vi "子界面-查看某框和报告生成.vi"(0 "框号":dbl format="%#_13g", 1 "框组":T4(array[cluster]), 2 "反射图":T1(plugin-control), 4 "标注图":T1(plugin-control)) -> ()   [LabVIEW 2018]
uses:
  <vilib>/vision/NI_Vision_Development_Module.lvlib
panel:
  out "反射图ROI对应区域灰度表":u32[](graph)
  out "报告生成路径":path
  out "?":T1(plugin-control)
  out "Threshold Image":T1(plugin-control)
  in  "格式字符串 2":string="%f"
  in  "分隔符（'\\'代码显示）":string="\t"
  out "分层测量结果":dbl[][](array[numeric]) format="%.2f"
  out "分层类检测结果":string[][](table)
  out "Threshold Image":T1(plugin-control)
  out "Threshold Image":T1(plugin-control)
  out "缺陷分类的临界值":sgl
  out "反射图ROI的最大灰度值":sgl
  in  "返回 2":bool
  in  "报告生成":bool
  in  "反射法图像-面积阈值设置":T3(array[cluster]) {"Measurement Parameter" items=["Area"]; "下限" min=0 step=1; "上限" min=0 step=1}
  in  "穿透法图像-灰度阈值设置":cluster{"下限":dbl, "下限":dbl}(slide)={"下限"=0.0, "下限"=65.10638427734375} scale=0.0..255.0
  in  "保存结果":bool
  in  "部位":string
  in  "Color":u32[](array[colorbox])=[3381759, 16776770, 16777225, 6618880]
  in  "Overlay Type":u16[](array[ring])=[2, 1, 3, 0] items=["Rectangle", "Numbers", "Points", "Lines"]
  in  "Tab Control":T5
  out "穿透ROI":T1(plugin-control)
  out "Threshold Image":T1(plugin-control)
  out "?":T1(plugin-control)
  out "?":T1(plugin-control)
  out "Threshold Image":T1(plugin-control)
  out "Threshold Image":T1(plugin-control)
  out "弥散测量结果":dbl[][](array[numeric]) format="%.2f"
  in  "产品序号":string
  in  "测试人":string
  in  "分隔符（'\\'代码显示）":string="\t"
  in  "格式字符串":string="%f"
  out "弥散类检测结果":string[][](table)
  out "?":string
  out "面积 (pixels)":i32
  # "所选区域信息"
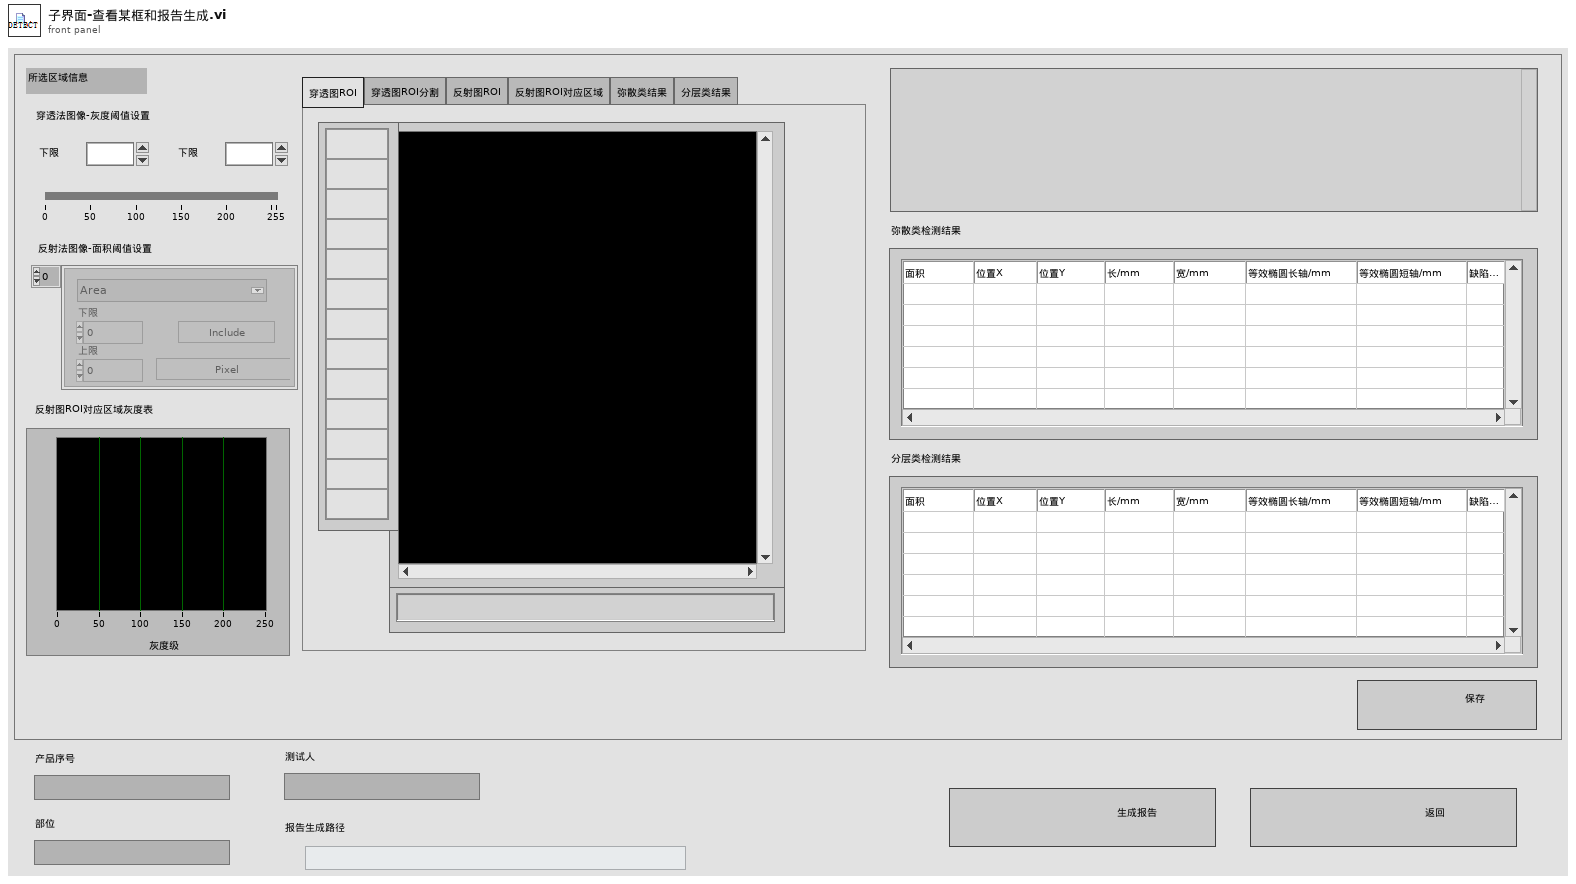
[diagram p1: front panel]
types:
  T1 = typedef "IMAQ Image.ctl" = refnum<image>
  T2 = typedef "Particle Parameters" = i32
  T3 = cluster{"Measurement Parameter":T2, "下限":i32, "上限":i32, "Range":bool, "Measurement Type":bool}[]
  T4 = cluster{"Global Rectangle":i32[], "Contours":cluster{"Contour Type":u32, "ROI Type":u32, "Points":i32[]}[]}[]
  T5 = typedef "控件11.ctl" = enum32{"穿透图ROI", "穿透图ROI分割", "反射图ROI", "反射图ROI对应区域", "弥散类结果", "分层类结果"}
  T6 = typedef "Image Type" = u32
  T7 = cluster{"Global Rectangle":i32[], "Contours":cluster{"Contour Type":u32, "ROI Type":u32, "Points":i32[]}[]}
  T8 = cluster{"Pixel Measurements":T2[], "Overlay Type":u16[], "Color":u32[], "反射法图像-面积阈值设置":cluster{"Measurement Parameter":T2, "下限":i32, "上限":i32, "Range":bool, "Measurement Type":bool}[], "穿透法图像-灰度阈值设置":cluster{"下限":dbl, "下限":dbl}}
  T9 = cluster{"histogram":u32[], "Minimal Value":sgl, "Maximal Value":sgl, "Starting Value":sgl, "Interval Width":sgl, "Mean Value":sgl, "Standard  Variation":sgl, "Area (pixels)":i32}
  T10 = cluster{"Desired Font (Application)":enum16{"User-specified Font", "Application Font", "System Font", "Dialog Font"}, "[User-specified Font]":cluster{"Font Name":string, "Size":i16, "Strikeout?":bool, "Italic?":bool, "Underline?":bool, "Outline?":bool, "Shadow?":bool, "Bold?":bool, "Rotation Angle":dbl}, "Horizontal Alignment":i16, "Vertical Alignment":i16}
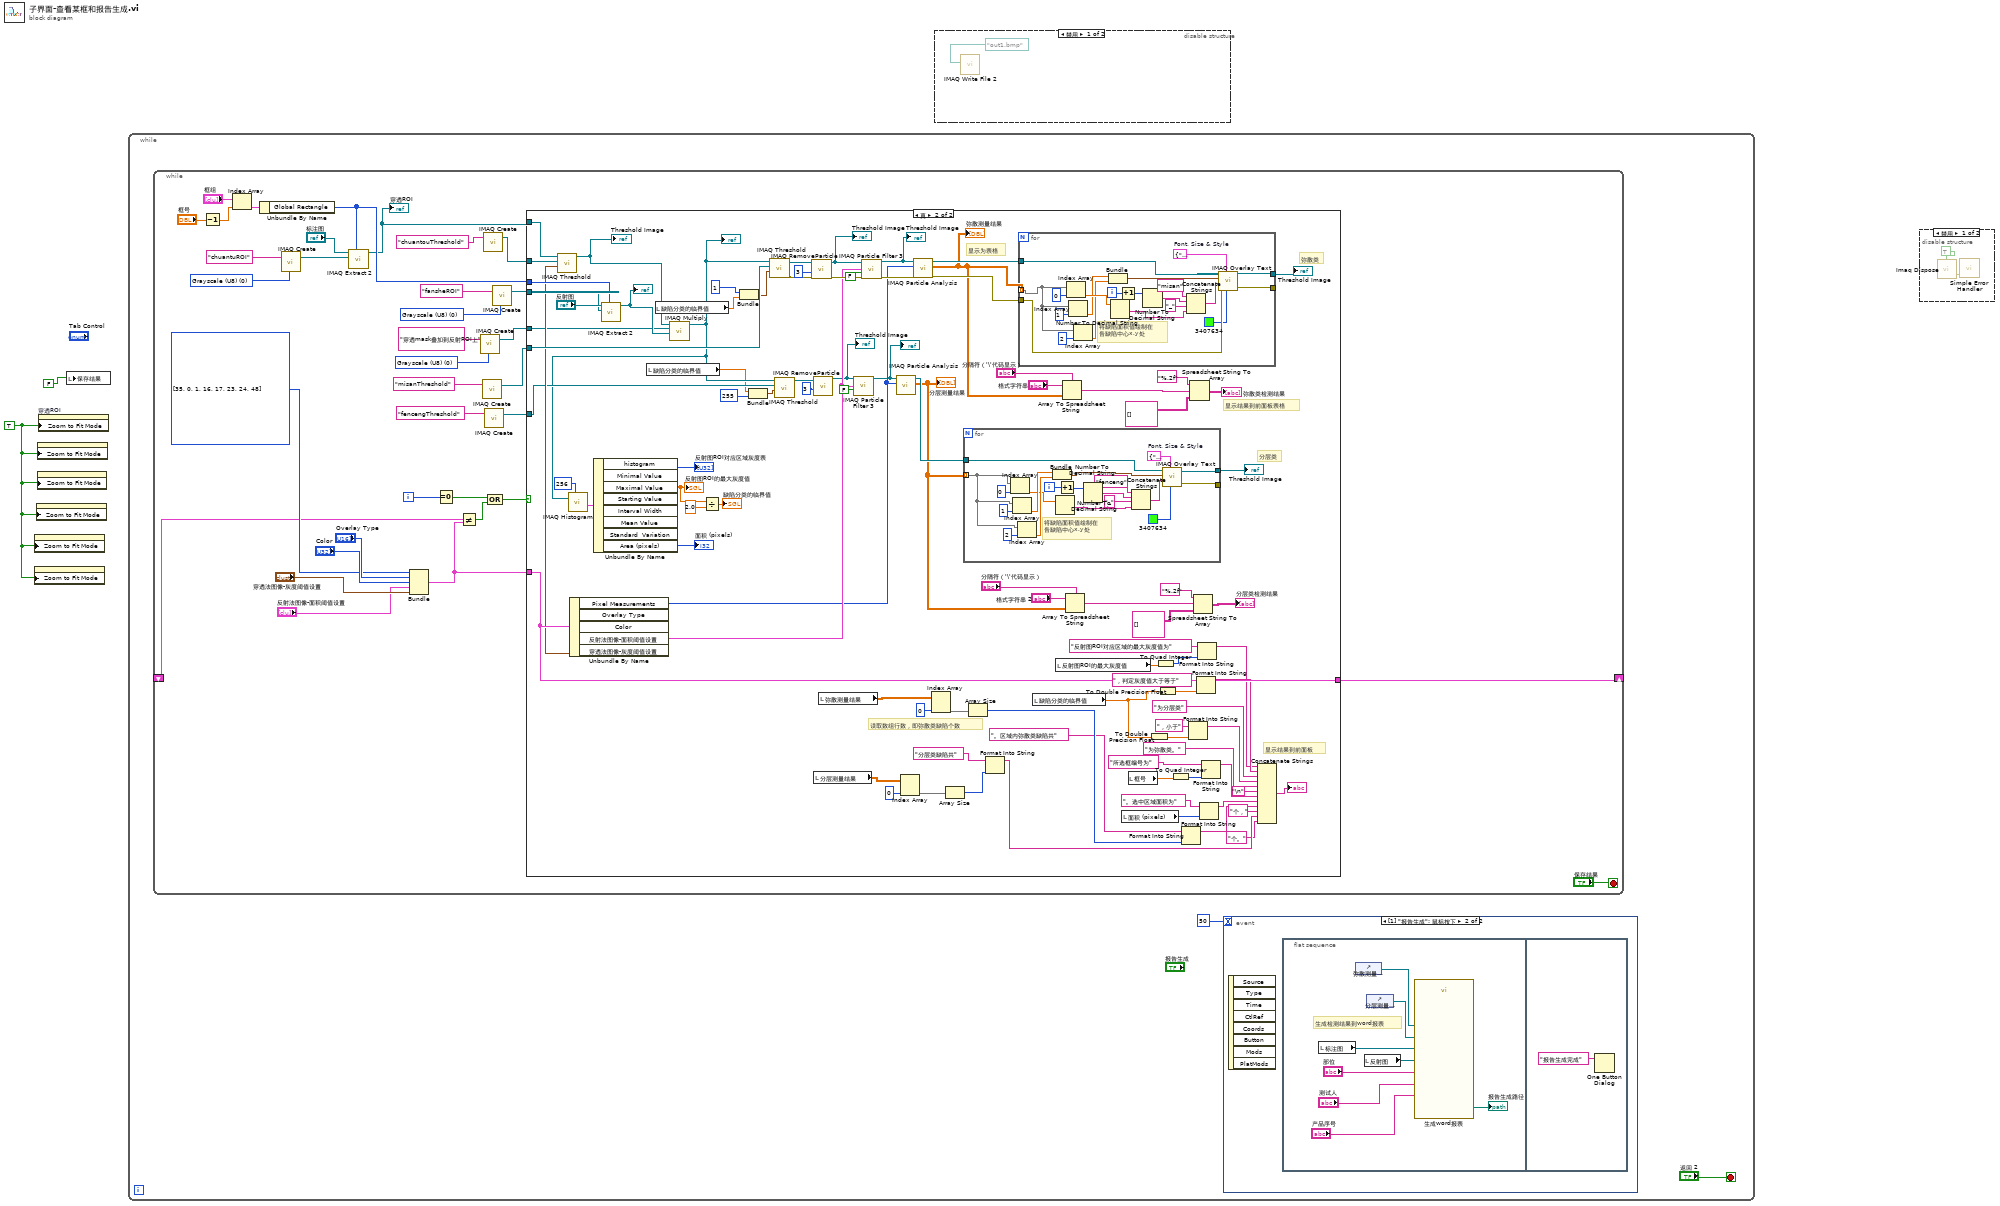
[diagram p0: block diagram]
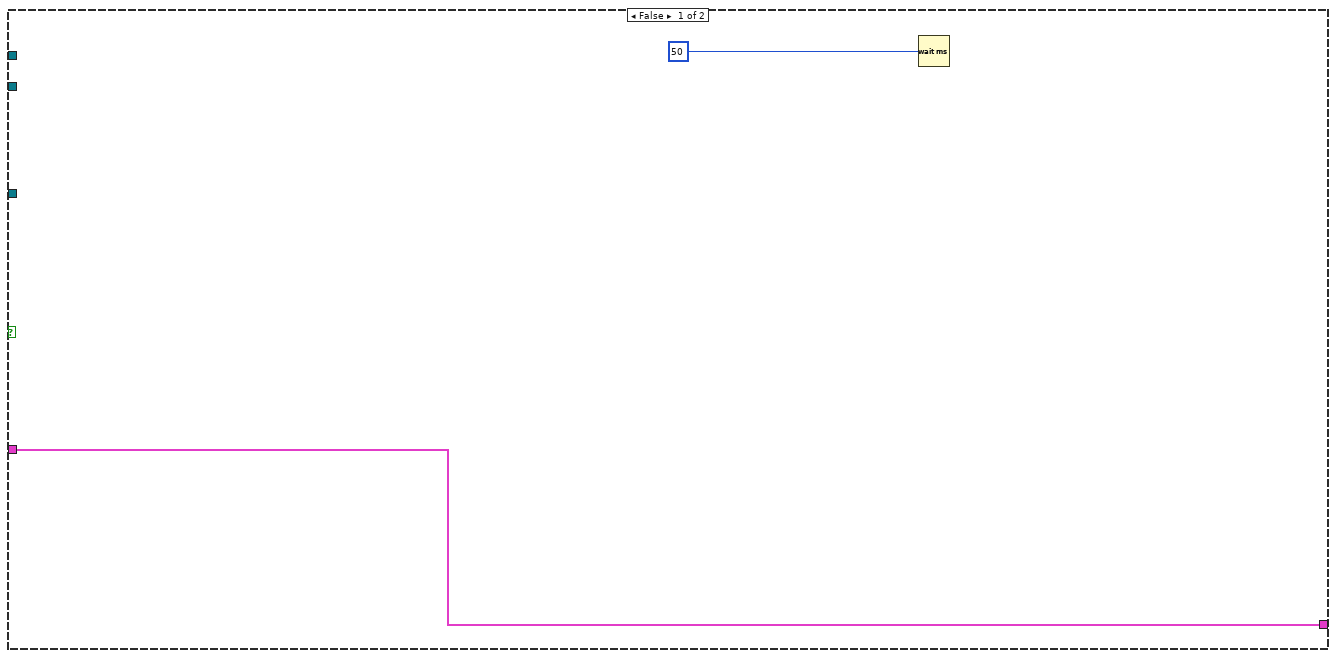
[diagram p3: hidden frame]
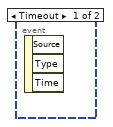
[diagram p4: hidden frame]
diagram:
  w1 = TRUE ("Zoom to Fit Mode")
  n1 = property class="ImageControl"("Zoom to Fit Mode"=w1) -> ()  [unwired: 2 in, 2 out]
  n2 = property class="ImageControl"("Zoom to Fit Mode"=w1) -> ()  [unwired: 2 in, 2 out]
  n3 = property class="ImageControl"("Zoom to Fit Mode"=w1) -> ()  [unwired: 2 in, 2 out]
  n4 = property class="ImageControl"("Zoom to Fit Mode"=w1) -> ()  [unwired: 2 in, 2 out]
  n5 = property class="ImageControl"("Zoom to Fit Mode"=w1) -> ()  [unwired: 2 in, 2 out]
  n6 = property on="穿透ROI" class="ImageControl"("Zoom to Fit Mode"=w1) -> ()  [unwired: 2 in, 2 out]
  n7 = local write "保存结果"(FALSE) -> ()
  n8 = while {
    stop <- "返回 2" stop-if-true
    n9 = while {
      shift-right: [w31] -> _
      shift-left: _ -> [w30]
      i -> [w35]
      stop <- "保存结果" stop-if-true
      w9 = T6 0 items=["Grayscale (U8)", "Grayscale (I16)", "Grayscale (SGL)", "Complex (CSG)", "RGB (U32)", "HSL (U32)", "RGB (U64)", "Grayscale (U16)"] ("Image Type")
      w16 = T6 0 items=["Grayscale (U8)", "Grayscale (I16)", "Grayscale (SGL)", "Complex (CSG)", "RGB (U32)", "HSL (U32)", "RGB (U64)", "Grayscale (U16)"] ("Image Type")
      w22 = T6 0 items=["Grayscale (U8)", "Grayscale (I16)", "Grayscale (SGL)", "Complex (CSG)", "RGB (U32)", "HSL (U32)", "RGB (U64)", "Grayscale (U16)"] ("Image Type")
      w37 = T2[] [35, 0, 1, 16, 17, 23, 24, 48] items=["Center of Mass X", "Center of Mass Y", "First Pixel X", "First Pixel Y", "Bounding Rect Left", "Bounding Rect Top", "Bounding Rect Right", "Bounding Rect Bottom", "Max Feret Diameter Start X", "Max Feret Diameter Start Y", "Max Feret Diameter End X", "Max Feret Diameter End Y", "Max Horiz. Segment Length Left", "Max Horiz. Segment Length Right", "Max Horiz. Segment Length Row", "-", "Bounding Rect Width", "Bounding Rect Height", "Bounding Rect Diagonal", "Perimeter", "Convex Hull Perimeter", "Holes' Perimeter", "Max Feret Diameter", "Equivalent Ellipse Major Axis", "Equivalent Ellipse Minor Axis", "Equivalent Ellipse Minor Axis (Feret)", "Equivalent Rect Long Side", "Equivalent Rect Short Side", "Equivalent Rect Diagonal", "Equivalent Rect Short Side (Feret)", "Average Horiz. Segment Length", "Average Vert. Segment Length", "Hydraulic Radius", "Waddel Disk Diameter", "-", "Area", "Holes' Area", "Particle & Holes' Area", "Convex Hull Area", "Image Area", "-", "Number of Holes", "Number of Horiz. Segments", "Number of Vert. Segments", "-", "Orientation", "Max Feret Diameter Orientation", "-", "% Area/Image Area", "% Area/(Particle & Holes' Area)", "Ratio of Equivalent Ellipse Axes", "Ratio of Equivalent Rect Sides", "-", "Elongation Factor", "Compactness Factor", "Heywood Circularity Factor", "Type Factor", "-", "Sum X", "Sum Y", "Sum XX", "Sum XY", "Sum YY", "Sum XXX", "Sum XXY", "Sum XYY", "Sum YYY", "-", "Moment of Inertia XX", "Moment of Inertia XY", "Moment of Inertia YY", "Moment of Inertia XXX", "Moment of Inertia XXY", "Moment of Inertia XYY", "Moment of Inertia YYY", "Norm. Moment of Inertia XX", "Norm. Moment of Inertia XY", "Norm. Moment of Inertia YY", "Norm. Moment of Inertia XXX", "Norm. Moment of Inertia XXY", "Norm. Moment of Inertia XYY", "Norm. Moment of Inertia YYY", "Hu Moment 1", "Hu Moment 2", "Hu Moment 3", "Hu Moment 4", "Hu Moment 5", "Hu Moment 6", "Hu Moment 7"] ("Pixel Measurements")
      n10 = Decrement(x="框号") -> (x-1=w24:dbl)
      n11 = Index Array(array="框组", index=w24) -> (element=w26:T7)
      n12 = Unbundle By Name(w26) -> ("Global Rectangle"=w14:i32[])
      n13 = call "IMAQ Create"("Image Name"="chuantuROI", "Image Type"=w22) -> ("New Image"=w25:T1)  [unwired: 3 in, 1 out]
      n14 = call "IMAQ Extract 2"("Optional Rectangle"=w14, "Image Dst"=w25, "Image Src"="标注图") -> ("Image Dst Out"=w12:T1)  [unwired: 7 in, 1 out]
      "穿透ROI" <- w12
      n15 = Bundle("Pixel Measurements"=w37, "Overlay Type"="Overlay Type", "Color"="Color", "反射法图像-面积阈值设置"="反射法图像-面积阈值设置", "穿透法图像-灰度阈值设置"="穿透法图像-灰度阈值设置") -> (w13:T8)  [unwired: 1 in]
      n16 = Equal To 0?(x=w35) -> (x = 0?=w34:bool)
      n17 = Not Equal?(x=w30, y=w13) -> (x != y?=w33:bool)
      n18 = call "IMAQ Create"("Image Name"="穿透mask叠加到反射ROI上", "Image Type"=w9) -> ("New Image"=w8:T1)  [unwired: 3 in, 1 out]
      n19 = call "IMAQ Create"("Image Name"="misanThreshold") -> ("New Image"=w7:T1)  [unwired: 4 in, 1 out]
      n20 = call "IMAQ Create"("Image Name"="chuantouThreshold") -> ("New Image"=w18:T1)  [unwired: 4 in, 1 out]
      n21 = call "IMAQ Create"("Image Name"="fencengThreshold") -> ("New Image"=w5:T1)  [unwired: 4 in, 1 out]
      n22 = Compound Arithmetic op=OR(w34, w33) -> (w32:bool)
      n23 = call "IMAQ Create"("Image Name"="fansheROI", "Image Type"=w16) -> ("New Image"=w15:T1)  [unwired: 3 in, 1 out]
      n24 = case shown="真" w32 {
        tunnel: w13 -> [w40 w103]
        tunnel: [w40 w103] -> w31
        tunnel: w18 -> [_ w111]
        tunnel: w12 -> [_ w101]
        tunnel: w15 -> [_ w109]
        tunnel: w14 -> [_ w108]
        tunnel: w7 -> [_ w107]
        tunnel: w8 -> [_ w98]
        tunnel: w5 -> [_ w70]
        frame False {
          n25 = Wait (ms)(milliseconds to wait=u32 50) -> ()  [unwired: 1 out]
        }
        frame True {
          # "分层类"
          # "弥散类"
          # "显示结果到前面板"
          # "读取数组行数，即弥散类缺陷个数"
          # "显示结果到前面板表格"
          # "显示为表格"
          n26 = Unbundle By Name(w103) -> ("Pixel Measurements"=w61:T2[], "反射法图像-面积阈值设置"=w63:T3, "穿透法图像-灰度阈值设置"=w102:cluster{"下限":dbl, "下限":dbl})  [unwired: 2 out]
          n27 = call "IMAQ Threshold"("Range"=w102, "Image Dst"=w111, "Image Src"=w101) -> ("Image Dst Out"=w100:T1)  [unwired: 3 in, 5 out]
          "Threshold Image" <- w100
          n28 = call "IMAQ Extract 2"("Optional Rectangle"=w108, "Image Dst"=w109, "Image Src"="反射图") -> ("Image Dst Out"=w99:T1)  [unwired: 7 in, 1 out]
          "?" <- w99
          n29 = local read "缺陷分类的临界值"() -> (w66:sgl)
          n30 = local read "缺陷分类的临界值"() -> (w77:sgl)
          n31 = call "IMAQ Multiply"("Image Src A"=w100, "Image Dst"=w98, "Image Src B"=w99) -> ("Image Dst Out"=w69:T1)  [unwired: 4 in, 1 out]
          "?" <- w69
          n32 = call "IMAQ Histogram"("Number of Classes"=256, "Image"=w69) -> ("Histogram Report"=w106:T9)  [unwired: 8 in, 1 out]
          n33 = Unbundle By Name(w106) -> ("histogram"=→"反射图ROI对应区域灰度表":u32[], "Maximal Value"=w94:sgl, "Area (pixels)"=→"面积 (pixels)":i32)  [unwired: 5 out]
          "反射图ROI的最大灰度值" <- w94
          n34 = Divide(x=w94, y=sgl 2.0) -> (x/y=→"缺陷分类的临界值":sgl)
          n35 = Bundle(1, "缺陷分类的临界值"=w77) -> (w76:cluster{i32, "缺陷分类的临界值":sgl})  [unwired: 1 in]
          n36 = Bundle("缺陷分类的临界值"=w66, 255) -> (w68:cluster{"缺陷分类的临界值":sgl, i32})  [unwired: 1 in]
          n37 = call "IMAQ Threshold"("Range"=w76, "Image Dst"=w107, "Image Src"=w69) -> ("error out"=w135:errorcluster, "Image Dst Out"=w112:T1)  [unwired: 3 in, 4 out]
          n38 = call "IMAQ Threshold"("Range"=w68, "Image Dst"=w70, "Image Src"=w69) -> ("Image Dst Out"=w65:T1)  [unwired: 3 in, 5 out]
          n39 = call "IMAQ RemoveParticle"("error in (no error)"=w135, "Number of Erosion"=3, "Image Src"=w112) -> ("error out"=w134:errorcluster, "Image Dst Out"=w74:T1)  [unwired: 7 in]
          "Threshold Image" <- w74
          n40 = local read "分层测量结果"() -> (w49:dbl[][])
          n41 = call "IMAQ RemoveParticle"("Number of Erosion"=3, "Image Src"=w65) -> ("Image Dst Out"=w44:T1)  [unwired: 8 in, 1 out]
          "Threshold Image" <- w44
          n42 = local read "弥散测量结果"() -> (w71:dbl[][])
          n43 = call "IMAQ Particle Filter 3"("Image Src"=w44, "Selection Values"=w63, "Keep/Remove Particles (F)"=FALSE) -> ("Image Dst Out"=w43:T1)  [unwired: 10 in, 2 out]
          "?" <- w43
          n44 = call "IMAQ Particle Filter 3"("Image Src"=w74, "Selection Values"=w63, "Keep/Remove Particles (F)"=FALSE, "error in (no error)"=w134) -> ("Image Dst Out"=w73:T1, "error out"=w133:errorcluster)  [unwired: 9 in, 1 out]
          "Threshold Image" <- w73
          n45 = call "IMAQ Particle Analysis"("Pixel Measurements"=w61, "Image"=w43) -> ("Particle Measurements (Pixels)"=w55:dbl[][], "Image Out (duplicate)"=w60:T1)  [unwired: 4 in, 4 out]
          "分层测量结果" <- w55
          n46 = Index Array(array=w49, index (col)=0 ("禁用的索引 (列)")) -> (element=w51:dbl[])  [unwired: 1 in]
          n47 = call "IMAQ Particle Analysis"("error in (no error)"=w133, "Pixel Measurements"=w61, "Image"=w73) -> ("error out"=w131:errorcluster, "Particle Measurements (Pixels)"=w113:dbl[][], "Image Out (duplicate)"=w132:T1)  [unwired: 3 in, 3 out]
          "弥散测量结果" <- w113
          n48 = Index Array(array=w71, index (col)=0 ("禁用的索引 (列)")) -> (element=w119:dbl[])  [unwired: 1 in]
          n49 = Array Size(array=w51) -> (size(s)=w47:i32)
          n50 = for {
            tunnel: [w157] -> _
            tunnel: [w156] -> w59
            tunnel: w60 -> [w143]
            tunnel: w55 -> [w141] mode=indexing
            i -> [w138]
            w154 = T10 {"Desired Font (Application)"=enum."Application Font", "[User-specified Font]"={"Font Name"="", "Size"=12, "Strikeout?"=FALSE, "Italic?"=FALSE, "Underline?"=FALSE, "Outline?"=FALSE, "Shadow?"=FALSE, "Bold?"=FALSE, "Rotation Angle"=0.0}, "Horizontal Alignment"=0, "Vertical Alignment"=0}  # Font, Size & Style
            # "将缺陷面积值绘制在\n各缺陷中心x,y处"
            n51 = Index Array(array=w141, index=0 ("索引")) -> (element=w140:dbl)
            n52 = Index Array(array=w141, index=1 ("索引")) -> (element=w151:dbl)
            n53 = Index Array(array=w141, index=2 ("索引")) -> (element=w149:dbl)
            n54 = Bundle("Numeric"=w151, "Numeric"=w149) -> (w142:cluster{"Numeric":dbl, "Numeric":dbl})  [unwired: 1 in]
            n55 = Number To Decimal String(number=w140) -> (decimal integer string=w146:string)  [unwired: 1 in]
            n56 = Increment(x=w138) -> (x+1=w139:i32)
            n57 = Number To Decimal String(number=w139) -> (decimal integer string=w148:string)  [unwired: 1 in]
            n58 = Concatenate Strings("fenceng" ("字符串"), w148, "_", w146) -> (w145:string)
            n59 = call "IMAQ Overlay Text"("Text Color (black)"=u32 3407634, "Font, Size & Style"=w154, "String"=w145, "Origin"=w142, "Image"=w143) -> ("error out"=w157:errorcluster, "Image Out"=w156:T1)  [unwired: 5 in]
          }
          "Threshold Image" <- w59
          n60 = Array Size(array=w119) -> (size(s)=w121:i32)
          n61 = Format Into String(initial string="分层类缺陷共" ("初始字符串"), w47) -> (resulting string=w46:string)  [unwired: 2 in, 1 out]
          n62 = for {
            tunnel: w131 -> [w178]
            tunnel: [w177] -> _
            tunnel: [w176] -> w75
            tunnel: w132 -> [w174]
            tunnel: w113 -> [w167] mode=indexing
            i -> [w159]
            w173 = T10 {"Desired Font (Application)"=enum."Application Font", "[User-specified Font]"={"Font Name"="", "Size"=12, "Strikeout?"=FALSE, "Italic?"=FALSE, "Underline?"=FALSE, "Outline?"=FALSE, "Shadow?"=FALSE, "Bold?"=FALSE, "Rotation Angle"=0.0}, "Horizontal Alignment"=0, "Vertical Alignment"=0}  # Font, Size & Style
            # "将缺陷面积值绘制在\n各缺陷中心x,y处"
            n63 = Index Array(array=w167, index=0 ("索引")) -> (element=w172:dbl)
            n64 = Index Array(array=w167, index=1 ("索引")) -> (element=w169:dbl)
            n65 = Index Array(array=w167, index=2 ("索引")) -> (element=w166:dbl)
            n66 = Bundle("Numeric"=w169, "Numeric"=w166) -> (w165:cluster{"Numeric":dbl, "Numeric":dbl})  [unwired: 1 in]
            n67 = Number To Decimal String(number=w172) -> (decimal integer string=w162:string)  [unwired: 1 in]
            n68 = Increment(x=w159) -> (x+1=w158:i32)
            n69 = Number To Decimal String(number=w158) -> (decimal integer string=w164:string)  [unwired: 1 in]
            n70 = Concatenate Strings("misan" ("字符串"), w164, "_", w162) -> (w161:string)
            n71 = call "IMAQ Overlay Text"("Text Color (black)"=u32 3407634, "Font, Size & Style"=w173, "error in (no error)"=w178, "String"=w161, "Origin"=w165, "Image"=w174) -> ("error out"=w177:errorcluster, "Image Out"=w176:T1)  [unwired: 4 in]
          }
          "Threshold Image" <- w75
          n72 = local read "缺陷分类的临界值"() -> (w87:sgl)
          n73 = local read "反射图ROI的最大灰度值"() -> (w97:sgl)
          n74 = Array To Spreadsheet String(delimiter (Tab)="分隔符（'\\'代码显示）", array=w113, 3:"格式字符串") -> (spreadsheet string=w127:string)
          n75 = Array To Spreadsheet String(delimiter (Tab)="分隔符（'\\'代码显示）", array=w55, 3:"格式字符串 2") -> (spreadsheet string=w54:string)
          n76 = local read "面积 (pixels)"() -> (w118:i32)
          n77 = local read "框号"() -> (w123:dbl)
          n78 = To Double Precision Float(number=w87) -> (double precision float=w89:dbl)
          n79 = To Quad Integer(1:w97) -> (0:w96:i64)
          n80 = To Double Precision Float(number=w87) -> (double precision float=w91:dbl)
          n81 = To Quad Integer(1:w123) -> (0:w122:i64)
          n82 = Format Into String(initial string="。区域内弥散类缺陷共" ("初始字符串"), w121) -> (resulting string=w80:string)  [unwired: 2 in, 1 out]
          n83 = Format Into String(initial string="，小于" ("初始字符串"), w89) -> (resulting string=w85:string)  [unwired: 2 in, 1 out]
          n84 = Spreadsheet String To Array(format string="%.2f", spreadsheet string=w127, array type (2D Dbl)=string[][] [] ("Array")) -> (array=→"弥散类检测结果":string[][])  [unwired: 1 in]
          n85 = Spreadsheet String To Array(format string="%.2f", spreadsheet string=w54, array type (2D Dbl)=string[][] [] ("Array")) -> (array=→"分层类检测结果":string[][])  [unwired: 1 in]
          n86 = Format Into String(initial string="，判定灰度值大于等于" ("初始字符串"), w91) -> (resulting string=w83:string)  [unwired: 2 in, 1 out]
          n87 = Format Into String(initial string="反射图ROI对应区域的最大灰度值为" ("初始字符串"), w96) -> (resulting string=w82:string)  [unwired: 2 in, 1 out]
          n88 = Format Into String(initial string="。选中区域面积为" ("字符串"), w118) -> (resulting string=w81:string)  [unwired: 2 in, 1 out]
          n89 = Format Into String(initial string="所选框编号为" ("初始字符串"), w122) -> (resulting string=w124:string)  [unwired: 2 in, 1 out]
          n90 = Concatenate Strings(w82, w83, "为分层类" ("初始字符串"), w85, "为弥散类。" ("初始字符串"), "\n", w124, w81, w80, "个，" ("字符串"), w46, "个。" ("字符串")) -> (→"?":string)
        }
      }
    }
    n91 = event shown="[1] \"报告生成\": 鼠标按下" {
      selector: _ -> [_ _]
      dyn-events: _ -> [_ _]
      timeout: 50 -> [_ _]
      event Timeout {
        n92 = event-data() -> ()  [unwired: 1 in, 3 out]
      }
      event "报告生成": Mouse Down {
        n93 = event-data() -> ()  [unwired: 1 in, 8 out]
        n94 = flat-sequence {
          frame #0 {
            # "生成检测结果到word报表"
            n95 = local read "标注图"() -> (w184:T1)
            n96 = control-ref of="弥散测量结果"() -> (w182:refnum<vi>)
            n97 = local read "反射图"() -> (w185:T1)
            n98 = control-ref of="分层测量结果"() -> (w181:refnum<vi>)
            n99 = call "生成word报表.vi"("Array输入"=w182, "产品序号"="产品序号", "标注图"=w185, "Array输入 2"=w181, "测试人"="测试人", "部位"="部位", "反射图"=w184) -> ("报告生成路径"=→"报告生成路径":path)  [unwired: 12 in]
          }
          frame #1 {
            n100 = One Button Dialog(message="报告生成完成" ("消息")) -> ()  [unwired: 1 in, 1 out]
          }
        }
      }
    }
  }
  n101 = disable-structure shown="禁用" {
    frame Disabled {
      n102 = call-poly "IMAQ Write File 2"("File Path"=path "out1.bmp") -> ()  [unwired: 9 in, 2 out]
    }
    frame Enabled {
    }
  }
  n103 = disable-structure shown="禁用" {
    frame Disabled {
      n104 = call "Imaq Dispose"("All Images? (No)"=TRUE) -> ("error out"=w190:errorcluster)  [unwired: 5 in]
      n105 = call <vilib>:"Simple Error Handler.vi"("error in (no error)"=w190) -> ()  [unwired: 4 in, 5 out]
    }
    frame Enabled {
    }
  }
